vi "Actor Core.vi"(8 "error in":errorcluster, 11 "Multimeter in":refnum<class "Multimeter.lvclass">) -> (0 "error out":errorcluster, 3 "Actor out":refnum<class "Actor.lvclass">)   [LabVIEW 2019, in "Multimeter.lvlib" / "Multimeter.lvclass"]
doc: "The instrument actor core is only here to distribute panel resolution settings to children classes."
uses:
  Library/Multimeter.lvclass
  C:/Users/Public/Documents/Development/builds/Instruments/Instruments.lvlibp/Library/Instruments.lvclass
  builds/Engine/Actor Framework.lvlibp/1abvi3w/vi.lib/ActorFramework/Actor/Actor.lvclass
  Custom Controls/Mode.ctl
  Library/Multimeter.lvclass/Multimeter.ctl
  Accessors/Write Table_Ref.vi
  builds/Instruments/Instruments.lvlibp/Accessors/Write Graph_Ref.vi
  builds/Instruments/Instruments.lvlibp/Library/Instruments.lvclass
panel:
  in  "Range":dbl=0.02
  in  "Mode":T1
  out "Waveform Chart":waveform(dbl)[](graph)
  out "Measured Table":i32(listbox)
  in  "Active Device":u16(ring)
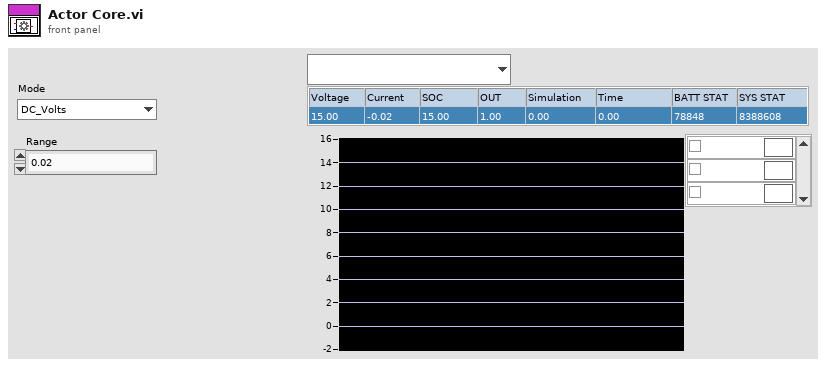
[diagram p1: front panel]
types:
  T1 = typedef "Multimeter.lvlib/Multimeter.lvclass/Mode.ctl" = enum16{"DC_Volts", "AC_Volts", "DC_Current", "AC_Current", "Resistance_2_Wire", "Resistance_4_Wire", "Diode", "Frequency", "Period", "AC_Volts_DC_Coupled", "Capacitance", "Inductance", "Temperature"}
  T2 = cluster{"Pnl Actor":refnum<event-registration>, "Event Registration Refnum":refnum<event-registration>}
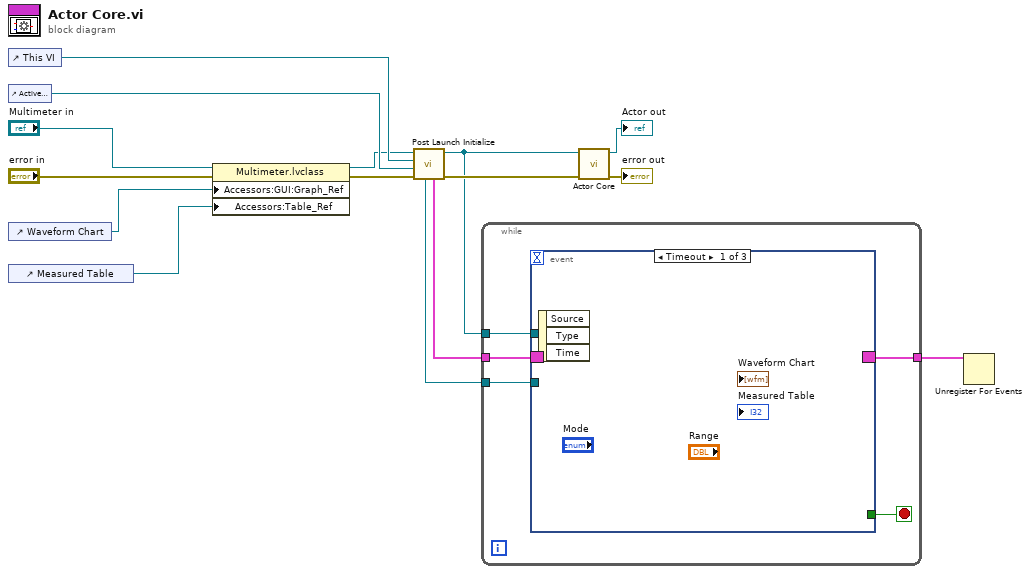
[diagram p0: block diagram]
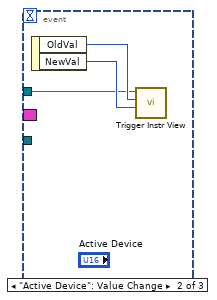
[diagram p2: hidden frame]
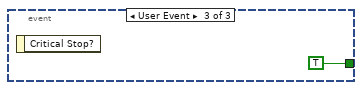
[diagram p3: hidden frame]
diagram:
  n1 = control-ref of="This VI"() -> (w10:refnum<vi>)
  n2 = control-ref of="Active Device"() -> (w9:refnum<vi>)
  n3 = control-ref of="Waveform Chart"() -> (w2:refnum<vi>)
  n4 = control-ref of="Measured Table"() -> (w1:refnum<vi>)
  n5 = property class="Multimeter.lvclass"(reference="Multimeter in", error in="error in", "Accessors:GUI:Graph_Ref"=w2, "Accessors:Table_Ref"=w1) -> (reference out=w6:refnum<class "Multimeter.lvclass">, error out=w5:errorcluster)
  n6 = call "Post Launch Initialize.vi"("error in"=w5, "Active Device"=w9, "GUI Reference"=w10, "Instruments in"=w6) -> ("error out"=w13:errorcluster, "Instruments out"=w8:refnum<class "Multimeter.lvclass">, "Registered Events"=w12:T2, "Self Enqueuer"=w11:refnum<class "Message Enqueuer.lvclass">)  [unwired: 4 in]
  n7 = while {
    tunnel: w12 -> [w20]
    tunnel: w11 -> [w19]
    tunnel: w8 -> [w18]
    tunnel: [w17] -> w7
    stop <- w16 stop-if-true
    n8 = event shown="[0] Timeout" {
      selector: w20 -> [_ _ _]
      dyn-events: [_ _ _] -> w17
      timeout: _ -> [_ _ _]
      tunnel: w19 -> [_ _ _]
      tunnel: w18 -> [_ w21 _]
      tunnel: [_ _ TRUE] -> w16
      event Timeout {
        n9 = event-data() -> ()  [unwired: 1 in, 3 out]
      }
      event "Active Device": Value Change {
        n10 = event-data() -> ("OldVal"=w23:u16, "NewVal"=w22:u16)  [unwired: 1 in]
        n11 = call "Trigger Instr View.vi"("New Value"=w22, "Old Value"=w23, "Instruments in"=w21) -> ()  [unwired: 7 in, 2 out]
      }
      event User Event {
        n12 = event-data() -> ()  [unwired: 1 in, 1 out]
      }
    }
  }
  n13 = call-parent "Actor Core.vi"("error in"=w13, "Instruments in"=w8) -> ("error out"=→"error out":errorcluster, "Actor out"=→"Actor out":refnum<class "Actor.lvclass">)  [unwired: 8 in]
  n14 = Unregister For Events(event registration refnum=w7) -> ()  [unwired: 1 in, 1 out]
